vi "Raw_To_Processed_Bytes.vi"(1 "Raw Bytes":u8[](array[numeric])) -> (0 "Processed Bytes":u8[](array[numeric]))   [LabVIEW 2017]
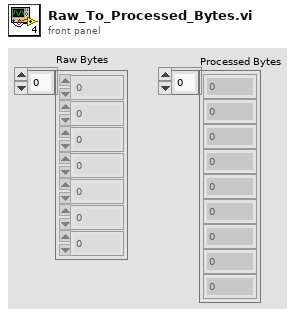
[diagram p1: front panel]
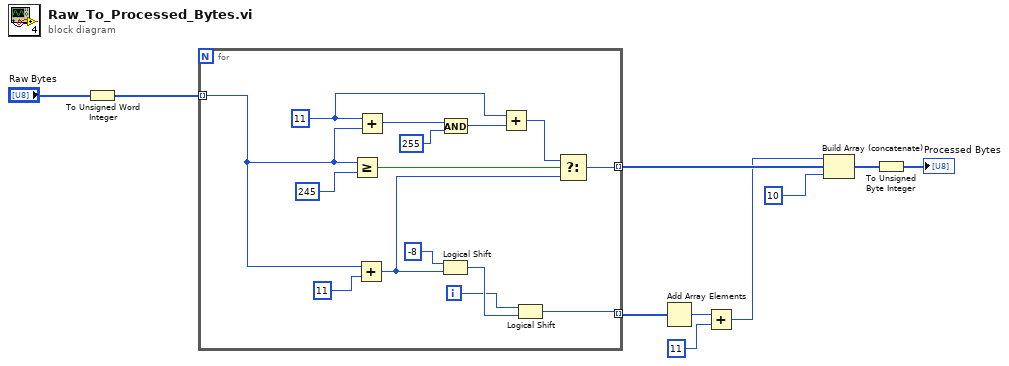
[diagram p0: block diagram]
diagram:
  n1 = To Unsigned Word Integer(number="Raw Bytes") -> (unsigned 16bit integer=w9:u16[])
  n2 = for {
    tunnel: w9 -> [w17] mode=indexing
    tunnel: [w18] -> w7 mode=indexing
    tunnel: [w12] -> w8 mode=indexing
    i -> [w13]
    w20 = u16 11 ("x")
    n3 = Greater Or Equal?(x=w17, y=u16 245) -> (x >= y?=w24:bool)
    n4 = Add(x=w17, y=u16 11) -> (x+y=w11:u16)
    n5 = Add(x=w20, y=w17) -> (x+y=w23:u16)
    n6 = Logical Shift(y=i16 -8, x=w11) -> (x << y=w14:u16)
    n7 = And(x=w23, y=u16 255) -> (x .and. y?=w21:u16)
    n8 = Add(x=w20, y=w21) -> (x+y=w19:u16)
    n9 = Logical Shift(y=w13, x=w14) -> (x << y=w12:u16)
    n10 = Select(t=w19, s=w24, f=w11) -> (s? t:f=w18:u16)
  }
  n11 = Add Array Elements(numeric array=w8) -> (sum=w3:u16)
  n12 = Add(x=w3, y=u16 11) -> (x+y=w2:u16)
  n13 = Build Array (concatenate)(w2, w7, u16 10) -> (w5:u16[])
  n14 = To Unsigned Byte Integer(number=w5) -> (unsigned 8bit integer=→"Processed Bytes":u8[])
